vi "SystemLink_Write_Number.vi"(9 "Numeric":dbl, 11 "SL_XControl":T1(xcontrol)) -> ()   [LabVIEW 2019]
uses:
  SL_XControl.xctl
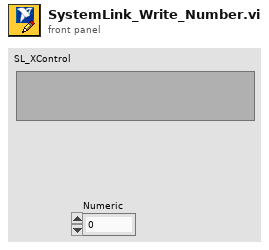
[diagram p1: front panel]
types:
  T1 = cluster{"Tag":string, "Type":string, "Data":string}
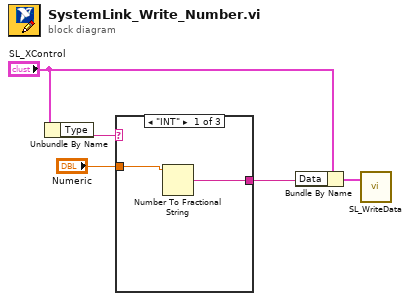
[diagram p0: block diagram]
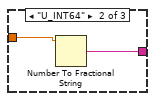
[diagram p2: hidden frame]
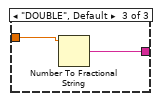
[diagram p3: hidden frame]
diagram:
  n1 = Unbundle By Name("SL_XControl") -> ("Type"=w4:string)
  n2 = case shown="\"INT\"" w4 {
    tunnel: "Numeric" -> [w7 w9 w11]
    tunnel: [w6 w8 w10] -> w3
    frame "INT" {
      n3 = Number To Fractional String(number=w7) -> (F-format string=w6:string)  [unwired: 3 in]
    }
    frame "U_INT64" {
      n4 = Number To Fractional String(number=w9) -> (F-format string=w8:string)  [unwired: 3 in]
    }
    frame "DOUBLE", Default {
      n5 = Number To Fractional String(number=w11) -> (F-format string=w10:string)  [unwired: 3 in]
    }
  }
  n6 = Bundle By Name(cluster="SL_XControl", "Data"=w3) -> (w1:T1)
  n7 = call "SL_WriteData.vi"("Tag"=w1) -> ()  [unwired: 11 in]
